vi "TAT-Load Reciepe data.vi"(8 "error in (no error)":errorcluster, 10 "Ref Data":T1 {"T-Bin Seq. Select"."First" max=8 step=1; "T-Bin Seq. Select"."Second" max=8 step=1; "T-Bin Seq. Select"."Third" max=8 step=1; "T-Bin Seq. Select"."Fourth" max=8 step=1; "T-Bin Seq. Select"."Fifth" max=8 step=1; "T-Bin Seq. Select"."Sixth" max=8; "Ass. Sensor Select"."Gun \nProg No." max=8 step=1; "Ass. Sensor Select"."Camera-2 \nProg No." max=8 step=1; "Ass. Sensor Select"."Camera-1 \nProg No." max=8 step=1}, 11 "Modbus Master in":refnum<class "Modbus Master.lvclass">) -> (0 "error out":errorcluster, 3 "Modbus Master out":refnum<class "Modbus Master.lvclass">)   [LabVIEW 2017]
uses:
  <vilib>/NI/Modbus Library/API/master/Modbus Master.lvclass
  Controls/Recipe.ctl
panel:
  # "Bin No."
  # "Bin No."
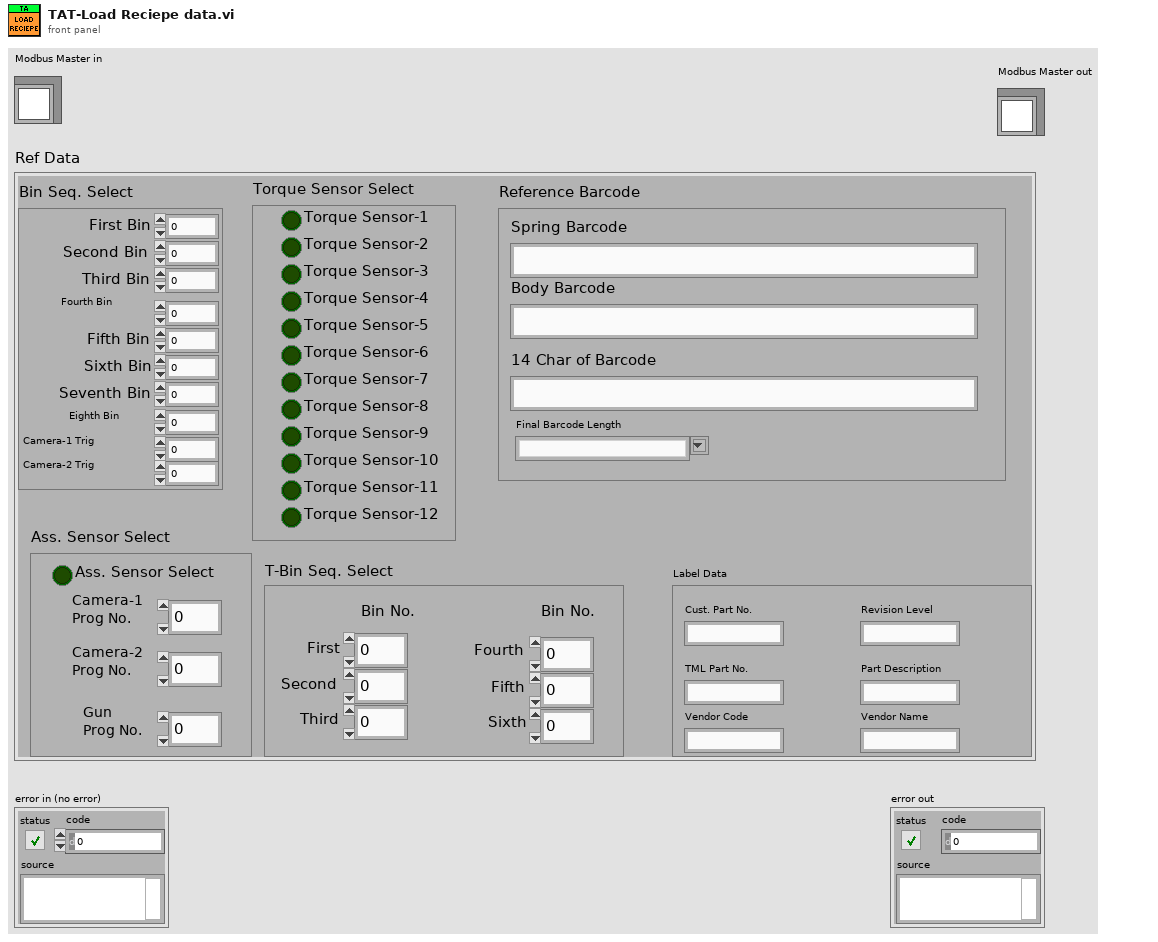
[diagram p1: front panel]
types:
  T1 = typedef "Recipe.ctl" = cluster{"Ass. Sensor Select":cluster{"Ass. Sensor Select":bool, "Camera-1 \nProg No.":u16, "Camera-2 \nProg No.":u16, "Gun \nProg No.":u16}, "Torque Sensor Select":cluster{"Torque Sensor-1":bool, "Torque Sensor-2":bool, "Torque Sensor-3":bool, "Torque Sensor-4":bool, "Torque Sensor-5":bool, "Torque Sensor-6":bool, "Torque Sensor-7":bool, "Torque Sensor-8":bool, "Torque Sensor-9":bool, "Torque Sensor-10":bool, "Torque Sensor-11":bool, "Torque Sensor-12":bool}, "Bin Seq. Select":cluster{"First Bin":u16, "Second Bin":u16, "Third Bin":u16, "Fourth Bin":u16, "Fifth Bin":u16, "Sixth Bin":u16, "Seventh Bin":u16, "Eighth Bin":u16, "Camera-1 Trig":u16, "Camera-2 Trig":u16}, "T-Bin Seq. Select":cluster{"First":u16, "Second":u16, "Third":u16, "Fourth":u16, "Fifth":u16, "Sixth":u16}, "Reference Barcode":cluster{"Spring Barcode":string, "Body Barcode":string, "14 Char of Barcode":string, "Final Barcode Length":string}, "Label Data":cluster{"Cust. Part No.":string, "TML Part No.":string, "Vendor Code":string, "Revision Level":string, "Part Description":string, "Vendor Name":string}}
  T2 = cluster{"First Bin":u16, "Second Bin":u16, "Third Bin":u16, "Fourth Bin":u16, "Fifth Bin":u16, "Sixth Bin":u16, "Seventh Bin":u16, "Eighth Bin":u16, "Camera-1 Trig":u16, "Camera-2 Trig":u16}
  T3 = cluster{"First":u16, "Second":u16, "Third":u16, "Fourth":u16, "Fifth":u16, "Sixth":u16}
  T4 = cluster{"Ass. Sensor Select":bool, "Camera-1 \nProg No.":u16, "Camera-2 \nProg No.":u16, "Gun \nProg No.":u16}
  T5 = cluster{"Torque Sensor-1":bool, "Torque Sensor-2":bool, "Torque Sensor-3":bool, "Torque Sensor-4":bool, "Torque Sensor-5":bool, "Torque Sensor-6":bool, "Torque Sensor-7":bool, "Torque Sensor-8":bool, "Torque Sensor-9":bool, "Torque Sensor-10":bool, "Torque Sensor-11":bool, "Torque Sensor-12":bool}
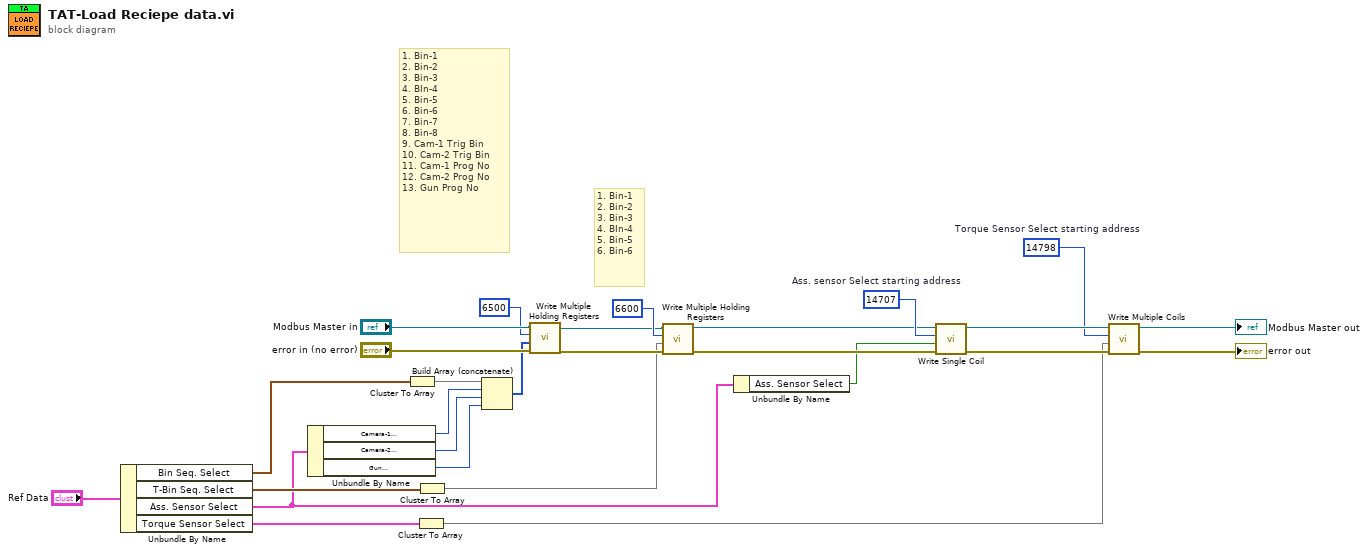
[diagram p0: block diagram]
diagram:
  w19 = u16 14798  # Torque Sensor Select starting address
  w21 = u16 14707  # Ass. sensor Select starting address
  # "1. Bin-1\n2. Bin-2\n3. Bin-3\n4. BIn-4\n5. Bin-5\n6. Bin-6"
  # "1. Bin-1\n2. Bin-2\n3. Bin-3\n4. BIn-4\n5. Bin-5\n6. Bin-6\n7. Bin-7\n8. Bin-8\n9. Cam-1 Trig Bin\n10. Cam-2 Trig Bin  \n11. Cam-1 Prog No\n12. Cam-2 Prog No\n13. Gun Prog No"
  n1 = Unbundle By Name("Ref Data") -> ("Bin Seq. Select"=w26:T2, "T-Bin Seq. Select"=w9:T3, "Ass. Sensor Select"=w7:T4, "Torque Sensor Select"=w10:T5)
  n2 = Unbundle By Name(w7) -> ("Camera-1 \nProg No."=w4:u16, "Camera-2 \nProg No."=w3:u16, "Gun \nProg No."=w1:u16)
  n3 = Cluster To Array(cluster=w26) -> (array=w6:u16[])
  n4 = Cluster To Array(cluster=w10) -> (array=w20:bool[])
  n5 = Cluster To Array(cluster=w9) -> (array=w8:u16[])
  n6 = Build Array (concatenate)(w6, w4, w3, w1) -> (w5:u16[])
  n7 = call-dynamic "Write Multiple Holding Registers.vi"("error in"="error in (no error)", "registers to write"=w5, "starting address"=u16 6500, "Modbus master in"="Modbus Master in") -> ("error out"=w13:errorcluster, "Modbus master out"=w14:refnum<class "Modbus Master.lvclass">)  [unwired: 6 in]
  n8 = call-dynamic "Write Multiple Holding Registers.vi"("error in"=w13, "registers to write"=w8, "starting address"=u16 6600, "Modbus master in"=w14) -> ("error out"=w11:errorcluster, "Modbus master out"=w12:refnum<class "Modbus Master.lvclass">)  [unwired: 6 in]
  n9 = Unbundle By Name(w7) -> ("Ass. Sensor Select"=w2:bool)
  n10 = call-dynamic "Write Single Coil.vi"("error in"=w11, "coil to write"=w2, "address"=w21, "Modbus master in"=w12) -> ("error out"=w23:errorcluster, "Modbus master out"=w25:refnum<class "Modbus Master.lvclass">)  [unwired: 6 in]
  n11 = call-dynamic "Write Multiple Coils.vi"("error in"=w23, "coils to write"=w20, "starting address"=w19, "Modbus master in"=w25) -> ("error out"=→"error out":errorcluster, "Modbus master out"=→"Modbus Master out":refnum<class "Modbus Master.lvclass">)  [unwired: 6 in]
